vi "New LINX-AutomationHat.vi"(8 "error in (no error)":errorcluster, 10 "Auto LED Control (T)":bool=TRUE, 11 "LINX Resource":T1={"IO"=enum."Remote", "Interface"=enum."Serial", "LINX Device Config"={"Interface"=enum."Serial", "COM Port"="COM13", "TCP Configuration"={"IP Address"="", "Port"=0}, "Device Family"=1, "Device ID"=1, "Device Name"="myRIO-1900", "TCP Ref"=refnum, "Channels"={"DI"=[0, 1, 2, 3, 4, 5, 6, 7, 8, 9, 10, 11, 12, 13, 14, 15, 16, 17, 18, 19, 20, 21, 22, 23, 24, 25, 26, 27, 28, 29, 30, 31, 32, 33, 34, 35, 36, 37, 38, 39, 40, 41, 42, 43, 44, 45, 46], "DO"=[0, 1, 2, 3, 4, 5, 6, 7, 8, 9, 10, 11, 12, 13, 14, 15, 16, 17, 18, 19, 20, 21, 22, 23, 24, 25, 26, 27, 28, 29, 30, 31, 32, 33, 34, 35, 36, 37, 38, 39, 40, 41, 42, 43, 44, 45, 46], "AI"=[0, 1, 2, 3, 4, 5, 6, 7, 8, 9, 10, 11], "AO"=[], "PWM"=[3, 5, 6, 9, 10], "QE"=[], "UART"=[0, 1], "I2C 2"=[0], "SPI"=[0], "CAN"=[], "Servo"=[], "AI Ref (V)"=0.0, "AI Resolution (Bits)"=0, "AO Ref (V)"=0.0, "AO Resolution (Bits)"=0}}}) -> (0 "error out":errorcluster, 3 "LINX-AutomationHat out":refnum<class "LINX-AutomationHat.lvclass">)   [LabVIEW 2020, in "LINX-AutomationHat.lvclass"]
uses:
  LINX-AutomationHat.lvclass
  <vilib>/MakerHub/LINX/Private/Type Defs/LINX Ref.ctl
  <vilib>/MakerHub/LINX/Private/Type Defs/Platform.ctl
  <vilib>/MakerHub/LINX/Private/Type Defs/Interface.ctl
  <vilib>/MakerHub/LINX/Private/Device/Type Defs/LINX Device Config.ctl
  <vilib>/MakerHub/LINX/Private/Device/Type Defs/TCP Config.ctl
  <vilib>/MakerHub/LINX/Private/Device/Type Defs/Channels.ctl
  LINX-ADS1015/ADC Type Selection.ctl
  LINX-ADS1015/Programmable Gain Selection.ctl
  LINX-ADS1015/ADS1015 Sample Rate.ctl
  LINX I2C/LINX I2C.lvclass
  LINX-ADS1015/LINX-ADS1X15.lvclass
  LINX-SN3218/LINX-SN3218.lvclass
  GPIO/LINX GPIO.lvclass
  <vilib>/MakerHub/LINX/LMH-LINX.lvlib
  <vilib>/MakerHub/LINX/Private/Device/Device.lvlib
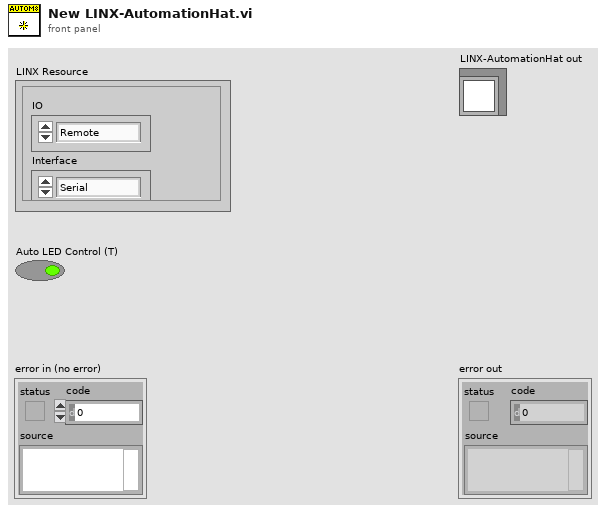
[diagram p1: front panel]
types:
  T1 = typedef "LMH-LINX.lvlib/LINX Ref.ctl" = cluster{"IO":T2, "Interface":T3, "LINX Device Config":T4}
  T2 = typedef "LMH-LINX.lvlib/Platform.ctl" = enum16{"Remote", "Local"}
  T3 = typedef "LMH-LINX.lvlib/Interface.ctl" = enum16{"Serial", "TCP"}
  T4 = typedef "LMH-LINX.lvlib/Device.lvlib/LINX Device Config.ctl" = cluster{"Interface":T3, "COM Port":refnum<visa-resource-name>, "TCP Configuration":T5, "Device Family":u8, "Device ID":u8, "Device Name":string, "TCP Ref":refnum<k5>, "Channels":T6}
  T5 = typedef "LMH-LINX.lvlib/Device.lvlib/TCP Config.ctl" = cluster{"IP Address":string, "Port":u16}
  T6 = typedef "LMH-LINX.lvlib/Channels.ctl" = cluster{"DI":u8[], "DO":u8[], "AI":u8[], "AO":u8[], "PWM":u8[], "QE":u8[], "UART":u8[], "I2C 2":u8[], "SPI":u8[], "CAN":u8[], "Servo":u8[], "AI Ref (V)":dbl, "AI Resolution (Bits)":u8, "AO Ref (V)":dbl, "AO Resolution (Bits)":u8}
  T7 = typedef "LINX-ADS1X15.lvclass/ADS1015 Sample Rate.ctl" = u16
  T8 = typedef "LINX-ADS1X15.lvclass/Programmable Gain Selection.ctl" = enum16{"+/-6.144V (2/3)", "+/-4.096V (1)", "+/-2.048V (2)", "+/-1.024V (4)", "+/-0.512V (8)", "+/-0.256V (16)"}
  T9 = typedef "LINX-ADS1X15.lvclass/ADC Type Selection.ctl" = enum16{"ADS1015", "ADS1115"}
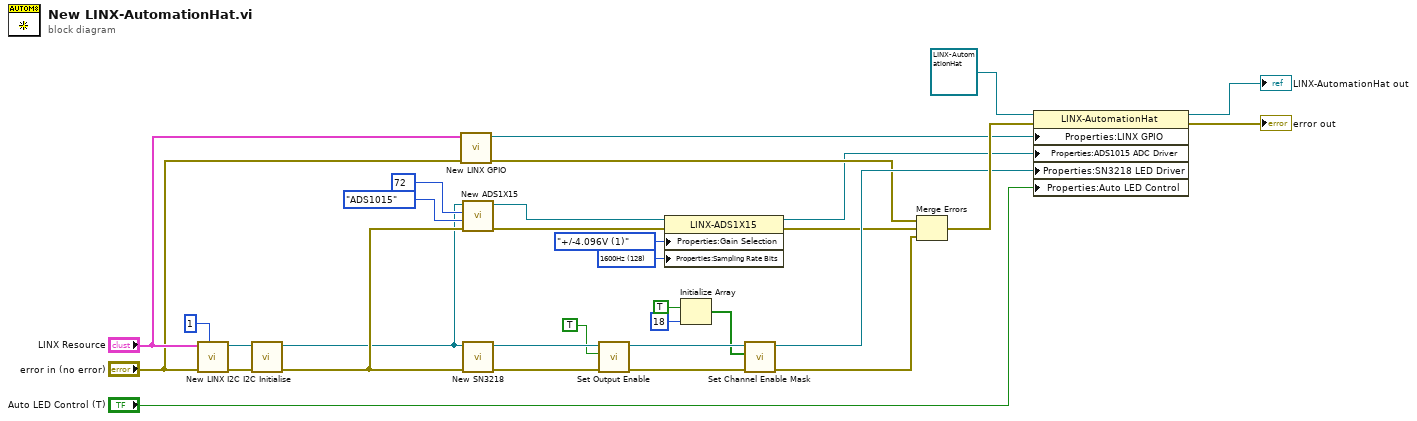
[diagram p0: block diagram]
diagram:
  w1 = T7 128 items=["128Hz"=0, "250Hz"=32, "490Hz"=64, "920Hz"=96, "1600Hz"=128, "2400Hz"=160, "3300Hz"=192] ("ADS1015 Sample Rate")
  n1 = call "New LINX I2C.vi"("LINX I2C Channel"=u8 1, "error in (no error)"="error in (no error)", "LINX Resource"="LINX Resource") -> ("error out"=w12:errorcluster, "LINX I2C out"=w11:refnum<class "LINX I2C.lvclass">)  [unwired: 7 in]
  n2 = call-dynamic "I2C Initialise.vi"("error in (no error)"=w12, "LINX I2C in"=w11) -> ("error out"=w10:errorcluster, "LINX I2C out"=w9:refnum<class "LINX I2C.lvclass">)  [unwired: 8 in]
  n3 = call "New LINX GPIO.vi"("error in (no error)"="error in (no error)", "LINX Resource"="LINX Resource") -> ("error out"=w14:errorcluster, "GPIO out"=w13:refnum<class "LINX GPIO.lvclass">)  [unwired: 8 in]
  n4 = call "New ADS1X15.vi"("error in (no error)"=w10, "ADC Type (ADS1015)"=ADC_Type_Selection."ADS1015", "I2C Slave Address (0x48)"=u8 72, "I2C"=w9) -> ("error out"=w4:errorcluster, "LINX-ADS1X15 out"=w29:refnum<class "LINX-ADS1X15.lvclass">)  [unwired: 6 in]
  n5 = call "New SN3218.vi"("error in (no error)"=w10, "I2C"=w9) -> ("error out"=w22:errorcluster, "LINX-SN3218 out"=w24:refnum<class "LINX-SN3218.lvclass">)  [unwired: 8 in]
  n6 = call "Set Output Enable.vi"("error in (no error)"=w22, "Enabled?"=TRUE, "LINX-SN3218 in"=w24) -> ("error out"=w17:errorcluster, "LINX-SN3218 out"=w21:refnum<class "LINX-SN3218.lvclass">)  [unwired: 7 in]
  n7 = property class="LINX-ADS1X15"(reference=w29, error in=w4, "Properties:Gain Selection"=Programmable_Gain_Selection."+/-4.096V (1)" ("Gain Selection"), "Properties:Sampling Rate Bits"=w1) -> (reference out=w5:refnum<class "LINX-ADS1X15.lvclass">, error out=w3:errorcluster)
  n8 = Initialize Array(TRUE, 18 ("dimension size")) -> (w18:bool[])
  n9 = call "Set Channel Enable Mask.vi"("error in (no error)"=w17, "Channel Enable"=w18, "LINX-SN3218 in"=w21) -> ("error out"=w15:errorcluster, "LINX-SN3218 out"=w16:refnum<class "LINX-SN3218.lvclass">)  [unwired: 7 in]
  n10 = Merge Errors(w14, w3, w15) -> (w27:errorcluster)
  n11 = property class="LINX-AutomationHat"(reference=refnum<class "LINX-AutomationHat.lvclass"> refnum ("LINX-AutomationHat in"), error in=w27, "Properties:LINX GPIO"=w13, "Properties:ADS1015 ADC Driver"=w5, "Properties:SN3218 LED Driver"=w16, "Properties:Auto LED Control"="Auto LED Control (T)") -> (reference out=→"LINX-AutomationHat out":refnum<class "LINX-AutomationHat.lvclass">, error out=→"error out":errorcluster)
